vi "ETH 4 Main.vi"(7 "ETH4 Q":refnum<queue>, 8 "error in (no error)":errorcluster, 10 "connection ID":refnum<k5>, 11 "data in":string) -> (0 "error out 2":errorcluster, 3 "connection ID 2":refnum<k5>)   [LabVIEW 2022 SP3]
panel:
  in  "ETH4 Q 2":refnum<queue>
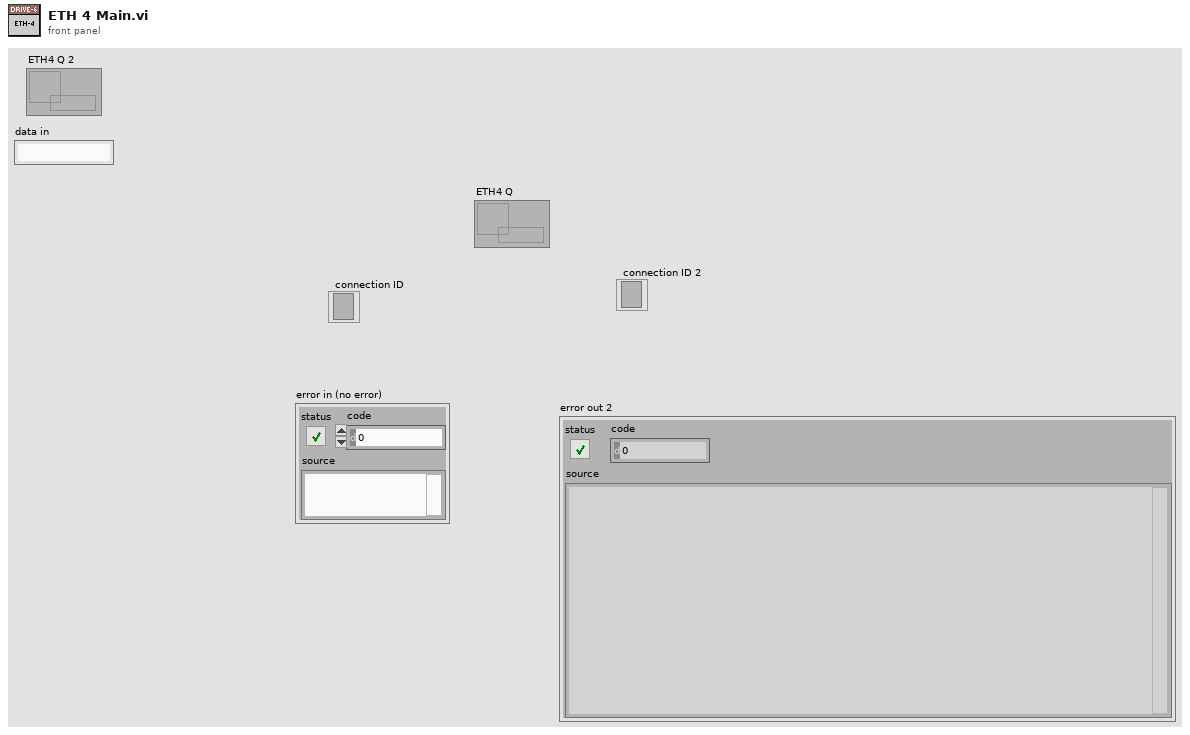
[diagram p1: front panel]
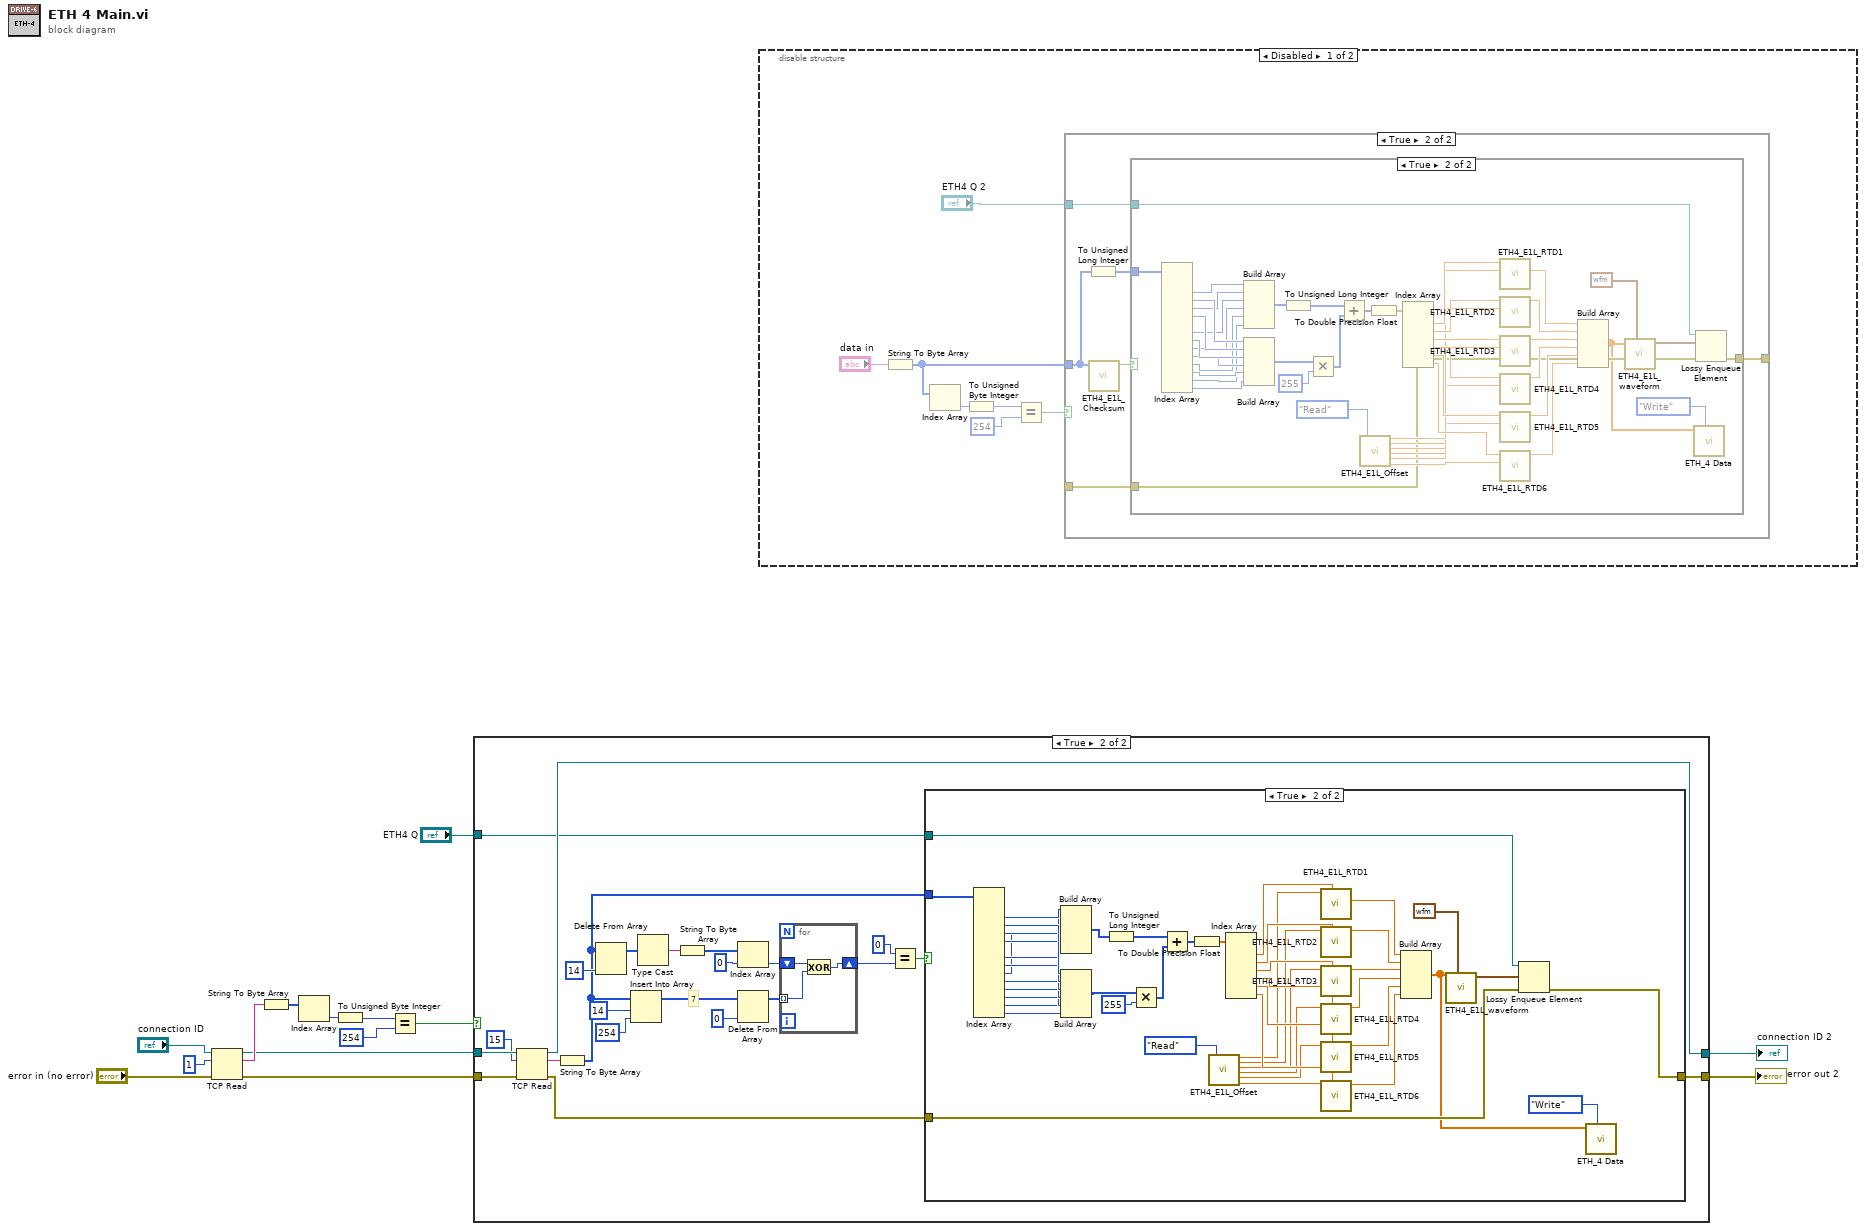
[diagram p0: block diagram]
diagram:
  n1 = TCP Read(connection ID="connection ID", bytes to read=1, error in (no error)="error in (no error)") -> (connection ID out=w8:refnum<k5>, data out=w9:string, error out=w6:errorcluster)  [unwired: 2 in]
  n2 = String To Byte Array(string=w9) -> (unsigned byte array=w13:u8[])
  n3 = Index Array(array=w13) -> (element=w12:u8)  [unwired: 1 in]
  n4 = To Unsigned Byte Integer(number=w12) -> (unsigned 8bit integer=w11:u8)
  n5 = Equal?(x=w11, y=u8 254) -> (x = y?=w7:bool)
  n6 = case shown="True" w7 {
    tunnel: w8 -> [w15 w39]
    tunnel: w6 -> [w16 w38]
    tunnel: [w16 w20] -> w4
    tunnel: [w15 w37] -> w3
    tunnel: "ETH4 Q" -> [_ w17]
    frame False {
    }
    frame True {
      # "7"
      n7 = TCP Read(connection ID=w39, bytes to read=15, error in (no error)=w38) -> (connection ID out=w37:refnum<k5>, data out=w36:string, error out=w19:errorcluster)  [unwired: 2 in]
      n8 = String To Byte Array(string=w36) -> (unsigned byte array=w18:u8[])
      n9 = Delete From Array(array=w18, index=14) -> (array with subset deleted=w27:u8[])  [unwired: 1 in, 1 out]
      n10 = Insert Into Array(array=w18, index=14, new element=u8 254 ("new element/subarray")) -> (w24:u8[])
      n11 = Type Cast(x=w27) -> (*(type *) &x=w33:string)  [unwired: 1 in]
      n12 = String To Byte Array(string=w33) -> (unsigned byte array=w28:u8[])
      n13 = Index Array(array=w28, index=0) -> (element=w31:u8)
      n14 = Delete From Array(array=w24, index=0) -> (array with subset deleted=w30:u8[])  [unwired: 1 in, 1 out]
      n15 = for {
        shift-right: [w88] -> w22
        shift-left: w31 -> [w89]
        tunnel: w30 -> [w87] mode=indexing
        n16 = Exclusive Or(1:w87, 2:w89) -> (0:w88:u8)
      }
      n17 = Equal?(x=u8 0, y=w22) -> (x = y?=w21:bool)
      n18 = case shown="True" w21 {
        tunnel: w18 -> [_ w78]
        tunnel: w17 -> [_ w81]
        tunnel: w19 -> [w40 w80]
        tunnel: [w40 w79] -> w20
        frame False {
        }
        frame True {
          n19 = Index Array(array=w78) -> (element #2=w75:u8, element #3=w74:u8, element #4=w73:u8, element #5=w72:u8, element #7=w71:u8, element #8=w70:u8, element #9=w69:u8, element #10=w68:u8, element #11=w67:u8, element #12=w66:u8, element #13=w65:u8, element #14=w64:u8)  [unwired: 14 in, 2 out]
          n20 = Build Array(w75, w73, w71, w69, w67, w65) -> (w77:u8[])
          n21 = Build Array(w74, w72, w70, w68, w66, w64) -> (w76:u8[])
          n22 = To Unsigned Long Integer(number=w77) -> (unsigned 32bit integer=w83:u32[])
          n23 = Multiply(x=w76, y=u32 255) -> (x*y=w85:u32[])
          n24 = Add(x=w83, y=w85) -> (x+y=w82:u32[])
          n25 = To Double Precision Float(number=w82) -> (double precision float=w86:dbl[])
          n26 = call "ETH4_E1L_Offset.vi"("Write/Read"=enum16{"Write", "Read"}."Read") -> ("RTD1 Offset Out"=w46:dbl, "RTD2 Offset Out"=w45:dbl, "RTD3 Offset Out"=w44:dbl, "RTD4 Offset out"=w43:dbl, "RTD5 Offset out"=w42:dbl, "RTD6 Offset  out"=w41:dbl)  [unwired: 13 in]
          n27 = Index Array(array=w86) -> (element #1=w54:dbl, element #2=w53:dbl, element #3=w52:dbl, element #4=w51:dbl, element #5=w50:dbl, element #6=w49:dbl)  [unwired: 6 in]
          n28 = call "ETH4_E1L_RTD1.vi"("Input Variable"=w54, "RTD 1 Off"=w46) -> ("RTD Value"=w60:dbl)  [unwired: 9 in]
          n29 = call "ETH4_E1L_RTD2.vi"("Input Variable"=w53, "RTD 2 Off"=w45) -> ("RTD Value"=w59:dbl)  [unwired: 9 in]
          n30 = call "ETH4_E1L_RTD3.vi"("Input Variable"=w52, "RTD 3 Off"=w44) -> ("RTD Value"=w58:dbl)  [unwired: 9 in]
          n31 = call "ETH4_E1L_RTD4.vi"("Input Variable"=w51, "RTD 4 Off"=w43) -> ("RTD Value"=w57:dbl)  [unwired: 9 in]
          n32 = call "ETH4_E1L_RTD5.vi"("Input Variable"=w50, "RTD 5 Off"=w42) -> ("RTD Value"=w56:dbl)  [unwired: 9 in]
          n33 = call "ETH4_E1L_RTD6.vi"("Input Variable"=w49, "RTD 6 Off"=w41) -> ("RTD Value"=w55:dbl)  [unwired: 9 in]
          n34 = Build Array(w60, w59, w58, w57, w56, w55) -> (w48:dbl[])
          n35 = call "ETH4_E1L_waveform.vi"("Waveform"=waveform(dbl) {"t0"=timestamp(0 s since 1904-01-01), "dt"=0.001, "Y"=[]}, "Array in"=w48) -> ("Array out"=w61:waveform(dbl)[])  [unwired: 9 in]
          n36 = Lossy Enqueue Element(queue=w81, element=w61, error in (no error)=w80) -> (error out=w79:errorcluster)  [unwired: 3 out]
          n37 = call "ETH_4 Data.vi"("Enum"=enum16{"Read", "Write"}."Write", "ETH_4"=w48) -> ()  [unwired: 8 in, 2 out]
        }
      }
    }
  }
  "error out 2" <- w4
  "connection ID 2" <- w3
  n38 = disable-structure shown="Disabled" {
    frame Disabled {
      n39 = String To Byte Array(string="data in") -> (unsigned byte array=w92:u8[])
      n40 = Index Array(array=w92) -> (element=w97:u8)  [unwired: 1 in]
      n41 = To Unsigned Byte Integer(number=w97) -> (unsigned 8bit integer=w96:u8)
      n42 = Equal?(x=w96, y=u8 254) -> (x = y?=w93:bool)
      n43 = case shown="True" w93 {
        tunnel: w92 -> [_ w103]
        tunnel: "ETH4 Q 2" -> [_ w101]
        tunnel: _ -> [w98 w100]
        tunnel: [w98 w99] -> w91
        frame False {
        }
        frame True {
          n44 = To Unsigned Long Integer(number=w103) -> (unsigned 32bit integer=w102:u32[])
          n45 = call "ETH4_E1L_Checksum.vi"("unsigned byte array"=w103) -> ("Checksum"=w104:bool)  [unwired: 10 in]
          n46 = case shown="True" w104 {
            tunnel: w102 -> [_ w120]
            tunnel: w101 -> [_ w126]
            tunnel: w100 -> [w105 w124]
            tunnel: [w105 w123] -> w99
            frame False {
            }
            frame True {
              n47 = Index Array(array=w120) -> (element #2=w117:u32, element #3=w116:u32, element #4=w115:u32, element #5=w114:u32, element #7=w113:u32, element #8=w112:u32, element #9=w111:u32, element #10=w110:u32, element #11=w109:u32, element #12=w108:u32, element #13=w107:u32, element #14=w106:u32)  [unwired: 14 in, 2 out]
              n48 = Build Array(w117, w115, w113, w111, w109, w107) -> (w119:u32[])
              n49 = Build Array(w116, w114, w112, w110, w108, w106) -> (w118:u32[])
              n50 = To Unsigned Long Integer(number=w119) -> (unsigned 32bit integer=w148:u32[])
              n51 = Multiply(x=w118, y=u32 255) -> (x*y=w150:u32[])
              n52 = Add(x=w148, y=w150) -> (x+y=w147:u32[])
              n53 = call "ETH4_E1L_Offset.vi"("Write/Read"=enum16{"Write", "Read"}."Read") -> ("RTD1 Offset Out"=w139:dbl, "RTD2 Offset Out"=w138:dbl, "RTD3 Offset Out"=w137:dbl, "RTD4 Offset out"=w136:dbl, "RTD5 Offset out"=w135:dbl, "RTD6 Offset  out"=w134:dbl)  [unwired: 13 in]
              n54 = To Double Precision Float(number=w147) -> (double precision float=w151:dbl[])
              n55 = Index Array(array=w151) -> (element #1=w146:dbl, element #2=w145:dbl, element #3=w144:dbl, element #4=w143:dbl, element #5=w142:dbl, element #6=w141:dbl)  [unwired: 6 in]
              n56 = call "ETH4_E1L_RTD1.vi"(10:w139, "RTD 1 Off"=w146) -> ("RTD Value"=w133:dbl)  [unwired: 9 in]
              n57 = call "ETH4_E1L_RTD2.vi"(10:w138, "RTD 2 Off"=w145) -> ("RTD Value"=w132:dbl)  [unwired: 9 in]
              n58 = call "ETH4_E1L_RTD3.vi"(10:w137, "RTD 3 Off"=w144) -> ("RTD Value"=w131:dbl)  [unwired: 9 in]
              n59 = call "ETH4_E1L_RTD4.vi"(10:w136, "RTD 4 Off"=w143) -> ("RTD Value"=w130:dbl)  [unwired: 9 in]
              n60 = call "ETH4_E1L_RTD5.vi"(10:w135, "RTD 5 Off"=w142) -> ("RTD Value"=w129:dbl)  [unwired: 9 in]
              n61 = call "ETH4_E1L_RTD6.vi"(10:w134, "RTD 6 Off"=w141) -> ("RTD Value"=w128:dbl)  [unwired: 9 in]
              n62 = Build Array(w133, w132, w131, w130, w129, w128) -> (w121:dbl[])
              n63 = call "ETH4_E1L_waveform.vi"("Waveform"=waveform(dbl) {"t0"=timestamp(0 s since 1904-01-01), "dt"=0.001, "Y"=[]}, "Array in"=w121) -> ("Array out"=w125:waveform(dbl)[])  [unwired: 9 in]
              n64 = call "ETH_4 Data.vi"("Enum"=enum16{"Read", "Write"}."Write", "ETH_4"=w121) -> ()  [unwired: 8 in, 2 out]
              n65 = Lossy Enqueue Element(queue=w126, element=w125, error in (no error)=w124) -> (error out=w123:errorcluster)  [unwired: 3 out]
            }
          }
        }
      }
    }
    frame Enabled {
    }
  }
